vi "CFTS-Read Defaults.vi"(0 "AppName":string="CFTS\\CAPTH", 2 "Type of anything":variant, 7 "User":string, 11 "error in (no error)":errorcluster) -> (4 "Anything":variant, 8 "Found?":bool, 15 "error out":errorcluster)   [LabVIEW 2020]
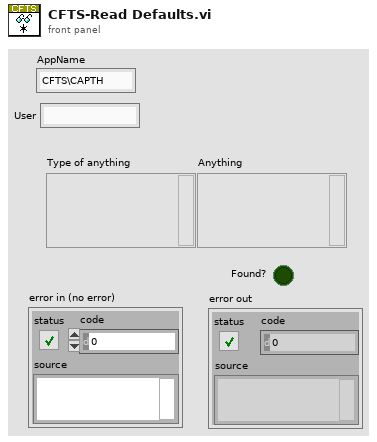
[diagram p1: front panel]
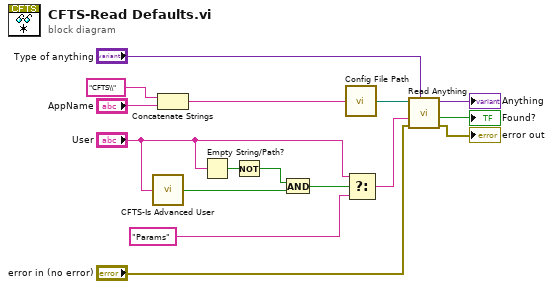
[diagram p0: block diagram]
diagram:
  n1 = call "CFTS-Is Advanced User.vi"("Experimenter"="User") -> ("Advanced user"=w10:bool)
  n2 = Concatenate Strings("CFTS\\" ("string"), "AppName") -> (w13:string)
  n3 = Empty String/Path?(string/path="User") -> (empty?=w2:bool)
  n4 = Not(x=w2) -> (.not. x?=w1:bool)
  n5 = And(x=w1, y=w10) -> (x .and. y?=w3:bool)
  n6 = call "Config File Path.vi"("AppName"=w13) -> ("Default config file name"=w16:path)
  n7 = Select(t="User", s=w3, f="Params") -> (s? t:f=w8:string)
  n8 = call "Read Anything.vi"("Type of Anything"="Type of anything", "Error In"="error in (no error)", "Section Name (Name of \"Type of Anything\")"=w8, "Path (dialog)"=w16) -> ("Error Out"=→"error out":errorcluster, "Found?"=→"Found?":bool, "Anything"=→"Anything":variant)  [unwired: 5 in]
